vi "读触发信息-触发不同拍照流程.vi"(8 "从PLC读取信息":T1 {"Mark拍照点坐标"."X" format="%#.3f"}, 11 "IO触发上升沿":T3) -> (1 "结束录视频":bool, 3 "7触发上位机读锁附结果":bool)   [LabVIEW 2014]
uses:
  Controls/XYPos.ctl
  Controls/MsgAction.ctl
panel:
  out "7触发上位机读锁附结果 2":bool
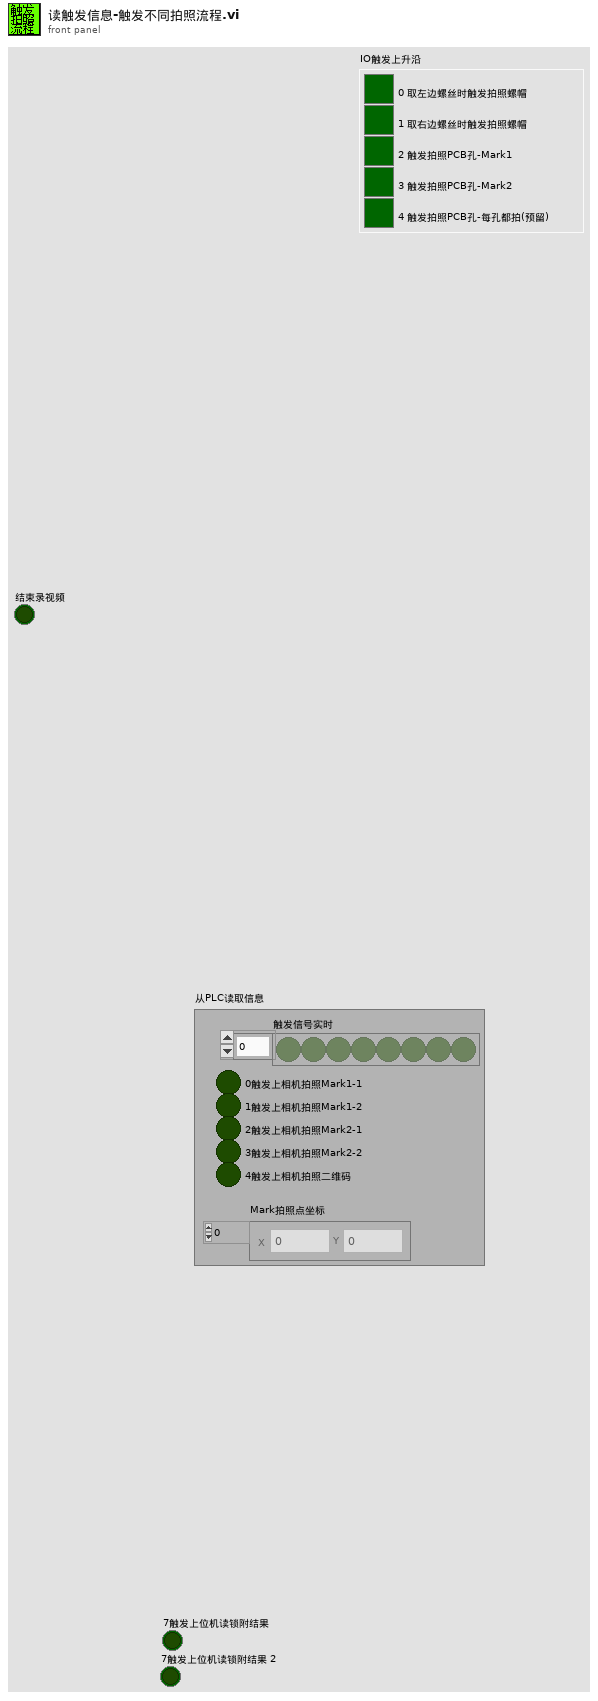
[diagram p1: front panel]
types:
  T1 = typedef "控件-UDP从PLC读取信息.ctl" = cluster{"触发信号实时":bool[], "0触发上相机拍照Mark1-1":bool, "1触发上相机拍照Mark1-2":bool, "2触发上相机拍照Mark2-1":bool, "3触发上相机拍照Mark2-2":bool, "4触发上相机拍照二维码":bool, "Mark拍照点坐标":T2[]}
  T2 = typedef "XYPos.ctl" = cluster{"X":dbl, "Y":dbl}
  T3 = cluster{"0 取左边螺丝时触发拍照螺帽":bool, "1 取右边螺丝时触发拍照螺帽":bool, "2 触发拍照PCB孔-Mark1":bool, "3 触发拍照PCB孔-Mark2":bool, "4 触发拍照PCB孔-每孔都拍(预留)":bool}
  T4 = typedef "MsgAction.ctl" = enum16{"初始化", "添加消息", "区分结果添加消息", "清空消息", "获取消息"}
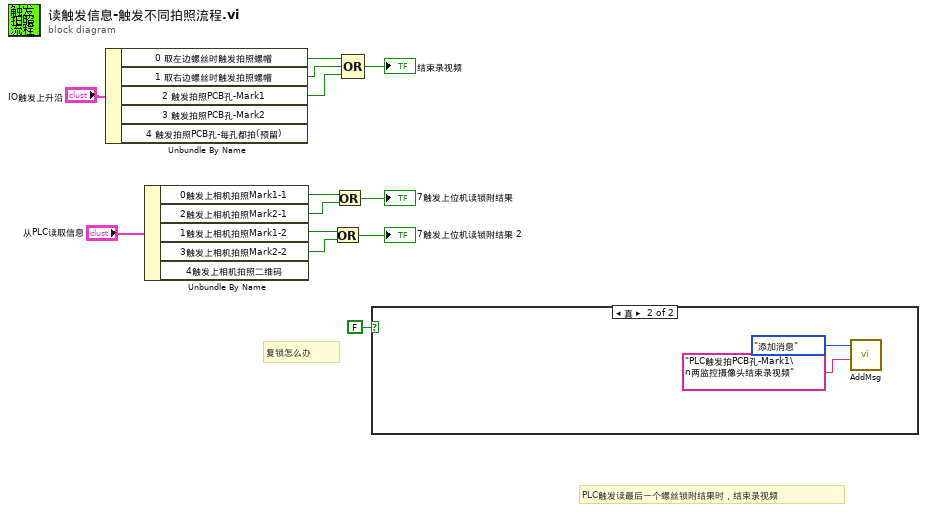
[diagram p0: block diagram]
diagram:
  # "复锁怎么办"
  # "PLC触发读最后一个螺丝锁附结果时，结束录视频"
  n1 = Unbundle By Name("IO触发上升沿") -> ("0 取左边螺丝时触发拍照螺帽"=w12:bool, "1 取右边螺丝时触发拍照螺帽"=w11:bool, "2 触发拍照PCB孔-Mark1"=w10:bool)  [unwired: 2 out]
  n2 = Unbundle By Name("从PLC读取信息") -> ("0触发上相机拍照Mark1-1"=w8:bool, "2触发上相机拍照Mark2-1"=w7:bool, "1触发上相机拍照Mark1-2"=w4:bool, "3触发上相机拍照Mark2-2"=w3:bool)  [unwired: 1 out]
  n3 = Or(x=w4, y=w3) -> (x .or. y?=→"7触发上位机读锁附结果 2":bool)
  n4 = Or(x=w8, y=w7) -> (x .or. y?=→"7触发上位机读锁附结果":bool)
  n5 = Compound Arithmetic op=OR(w12, w11, w10) -> (→"结束录视频":bool)
  n6 = case shown="真" FALSE {
    frame False {
    }
    frame True {
      n7 = call "AddMsg.vi"("添加消息"="PLC触发拍PCB孔-Mark1\n两监控摄像头结束录视频" ("消息显示"), "消息Action"=MsgAction."添加消息") -> ()  [unwired: 2 in, 1 out]
    }
  }
